vi "TurretOutput.vi"() -> ()   [LabVIEW 2019]
uses:
  refnums.vi
  outputs.vi
  sensors.vi
  dsdata.vi
  GRNF_GenericMotor.vi
panel:
  in  "Plot Turret":bool
  out "Turret PID Error":cluster{"Goal Wheel Position":dbl, dbl}(graph)={"Goal Wheel Position"=0.0, -90.17571233858979}
  out "Turret PID Contribution":cluster{dbl, dbl, dbl}(graph)
  in  "Turret N-Int":i32=10 caption="N-Int"
  in  "Turret N-Diff":i32=10 caption="N-Diff"
  in  "Turret Kd":dbl
  in  "Turret Ki":dbl
  in  "Turret Kp":dbl
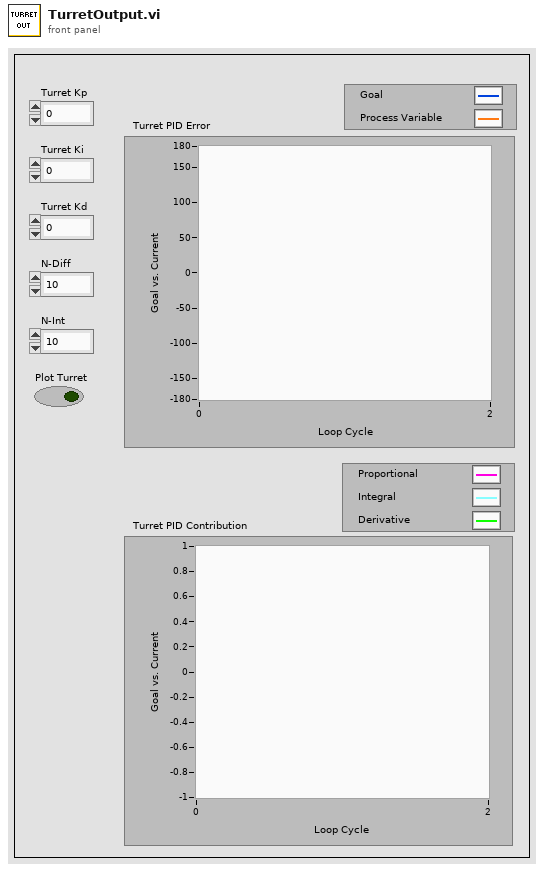
[diagram p1: front panel]
types:
  T1 = typedef "WPI_MotorControlDeviceRef.ctl" = cluster{"DeviceStatus":errorcluster, "Type":T2, "PWM":cluster{"PWM Channel":T3, "DeadBand":T4}, "CAN":cluster{"Device Number":u8, "SetOutput VI Ref":variant, "GetOutput VI Ref":variant, "Enable VI Ref":variant, "Disable VI Ref":variant, "Data":variant}, "Invert":bool, "DIO PWM":cluster{"PWM \"Enable\" Channel":T3, "DIOChannel":T5, "PWM Rate":dbl}}
  T2 = typedef "WPI_MotorControlType.ctl" = enum16{"PWM", "CAN", "DIO PWM"}
  T3 = typedef "FPGA_DIOPWMChannel.ctl" = enum8{"PWM 0", "PWM 1", "PWM 2", "PWM 3", "PWM 4", "PWM 5", "PWM 6", "PWM 7", "PWM 8", "PWM 9", "PWM MXP 0", "PWM MXP 1", "PWM MXP 2", "PWM MXP 3", "PWM MXP 4", "PWM MXP 5", "PWM MXP 6", "PWM MXP 7", "PWM MXP 8", "PWM MXP 9", "Invalid"}
  T4 = typedef "WPI_PWMDeadband.ctl" = cluster{"Name":string, "maxPositivePwm":i32, "minPositivePwm":i32, "centerPwm":i32, "maxNegativePwm":i32, "minNegativePwm":i32, "angularRange":u16}
  T5 = typedef "FPGA_DIOChannel.ctl" = enum8{"DIO 0", "DIO 1", "DIO 2", "DIO 3", "DIO 4", "DIO 5", "DIO 6", "DIO 7", "DIO 8", "DIO 9", "DIO MXP 0", "DIO MXP 1", "DIO MXP 2", "DIO MXP 3", "DIO MXP 4", "DIO MXP 5", "DIO MXP 6", "DIO MXP 7", "DIO MXP 8", "DIO MXP 9", "DIO MXP 10", "DIO MXP 11", "DIO MXP 12", "DIO MXP 13", "DIO MXP 14", "DIO MXP 15", "SPI Port CS1", "SPI Port CS2", "SPI Port CS3", "SPI Port MISO", "SPI Port MOSI", "Invalid"}
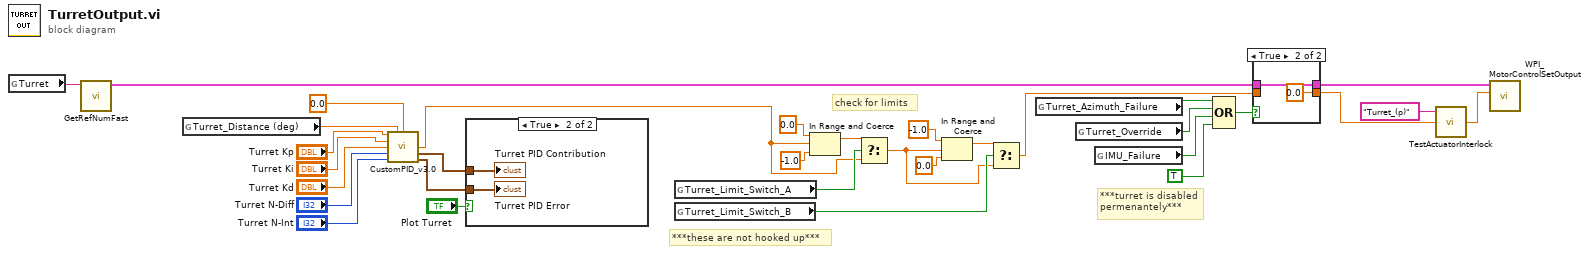
[diagram p0: block diagram]
diagram:
  # "***turret is disabled\npermenantely***"
  # "***these are not hooked up***"
  # "check for limits"
  n1 = global read "refnums.vi" "Turret"() -> (w1:string)
  n2 = call-poly "GetRefNumFast.vi"("RefNum Name"=w1) -> ("Device Reference"=w2:T1)  [unwired: 5 in, 1 out]
  n3 = global read "outputs.vi" "Turret_Distance (deg)"() -> (w3:dbl)
  n4 = call "CustomPID_v3.0.vi"("Kp"="Turret Kp", "Process Variable"=w3, "Goal"=0.0, "Ki"="Turret Ki", "Kd"="Turret Kd", "N-Diff"="Turret N-Diff", "N-Int"="Turret N-Int") -> ("Command"=w23:dbl, "Contribution Tracking"=w10:cluster{dbl, dbl, dbl}, "PID Tracking"=w11:cluster{"Goal Wheel Position":dbl, dbl})  [unwired: 5 in, 1 out]
  n5 = case shown="True" "Plot Turret" {
    tunnel: w10 -> [_ w34]
    tunnel: w11 -> [_ w33]
    frame False {
    }
    frame True {
      "Turret PID Contribution" <- w34
      "Turret PID Error" <- w33
    }
  }
  n6 = global read "sensors.vi" "Turret_Limit_Switch_A"() -> (w26:bool)
  n7 = global read "sensors.vi" "Turret_Limit_Switch_B"() -> (w27:bool)
  n8 = In Range and Coerce(upper limit=0.0, x=w23, lower limit=-1.0) -> (coerced(x)=w17:dbl)  [unwired: 1 out]
  n9 = Select(t=w17, s=w26, f=w23) -> (s? t:f=w24:dbl)
  n10 = In Range and Coerce(upper limit=-1.0, x=w24, lower limit=0.0) -> (coerced(x)=w20:dbl)  [unwired: 1 out]
  n11 = Select(t=w20, s=w27, f=w24) -> (s? t:f=w25:dbl)
  n12 = global read "sensors.vi" "Turret_Azimuth_Failure"() -> (w15:bool)
  n13 = global read "dsdata.vi" "Turret_Override"() -> (w16:bool)
  n14 = global read "sensors.vi" "IMU_Failure"() -> (w31:bool)
  n15 = Compound Arithmetic op=OR(w15, w16, w31, TRUE ("value")) -> (w14:bool)
  n16 = case shown="True" w14 {
    tunnel: [w36 w38] -> w13
    tunnel: w2 -> [w36 w38]
    tunnel: [w35 0.0 ("Command")] -> w29
    tunnel: w25 -> [w35 _]
    frame False {
    }
    frame True {
    }
  }
  n17 = call "TestActuatorInterlock.vi"("Input_Value_Double"=w29, "Actuator_Name"="Turret_(p)") -> ("Output_Value_Double"=w30:dbl)  [unwired: 1 in, 2 out]
  n18 = call <vilib>:"WPI_MotorControlSetOutput.vi"("Output"=w30, "MotorControlDevRef"=w13) -> ()  [unwired: 7 in, 3 out]
